vi "shopassert.vi"(8 "价格(小于等于） 2":dbl, 9 "名称 2":string, 10 "价格":dbl, 11 "食品名称":string) -> (1 "正确":bool, 2 "价格(小于等于） 3":dbl, 3 "名称 3":string)   [LabVIEW 2013, in "ShopBase.lvclass"]
uses:
  ShopBase.lvclass
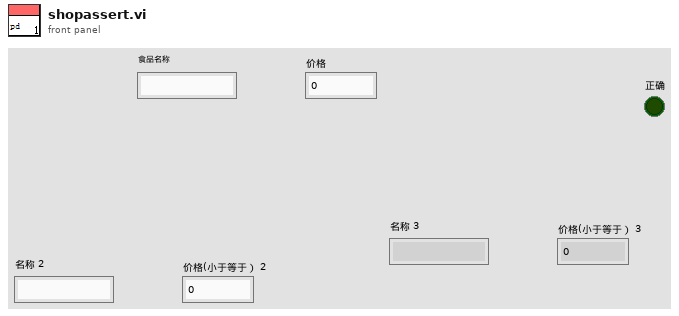
[diagram p1: front panel]
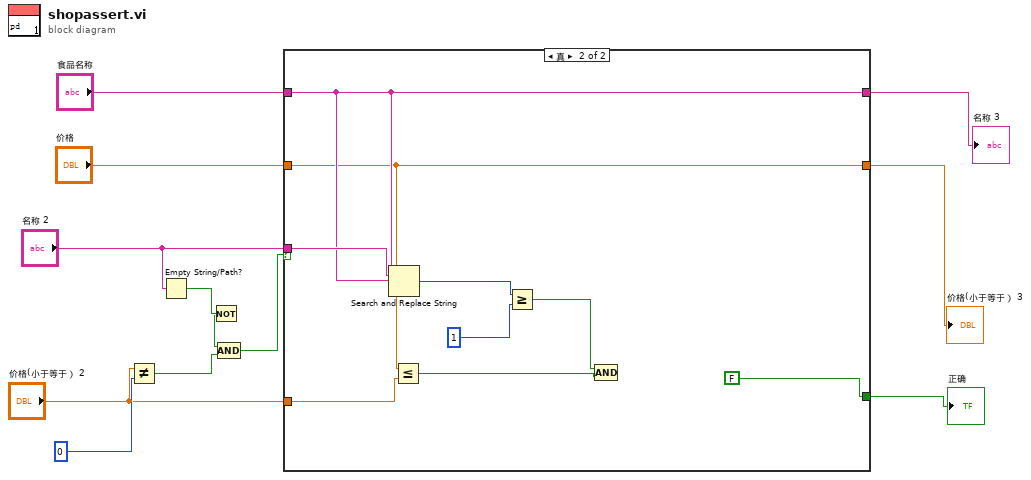
[diagram p0: block diagram]
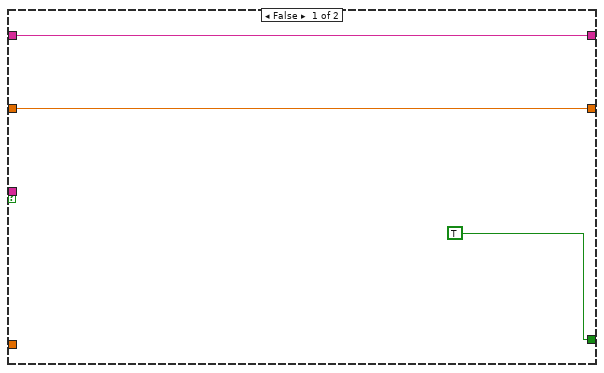
[diagram p2: hidden frame]
diagram:
  n1 = Not Equal?(x="价格(小于等于） 2", y=0) -> (x != y?=w11:bool)
  n2 = Empty String/Path?(string/path="名称 2") -> (empty?=w2:bool)
  n3 = Not(x=w2) -> (.not. x?=w1:bool)
  n4 = Compound Arithmetic op=AND(w1, w11) -> (w10:bool)
  n5 = case shown="真" w10 {
    tunnel: "食品名称" -> [w15 w18]
    tunnel: "价格" -> [w14 w17]
    tunnel: [w15 w18] -> w7
    tunnel: [w14 w17] -> w6
    tunnel: [TRUE FALSE] -> w5
    tunnel: "名称 2" -> [_ w24]
    tunnel: "价格(小于等于） 2" -> [_ w21]
    frame False {
    }
    frame True {
      n6 = Search and Replace String(input string=w18, search string=w24, replace string=w18) -> (number of replacements=w23:i32)  [unwired: 5 in, 3 out]
      n7 = Less Or Equal?(x=w17, y=w21) -> (x <= y?=w19:bool)
      n8 = Greater Or Equal?(x=w23, y=1) -> (x >= y?=w20:bool)
      n9 = Compound Arithmetic op=AND(w20, w19) -> ()  [unwired: 1 out]
    }
  }
  "名称 3" <- w7
  "价格(小于等于） 3" <- w6
  "正确" <- w5
